vi "Get Injected Value static.vi"(8 "error in (no error)":errorcluster, 11 "Fault-Injection_SGL in":refnum<class "Fault-Injection_SGL.lvclass">) -> (0 "error out":errorcluster, 2 "Value":T1, 3 "Fault-Injection_SGL out":refnum<class "Fault-Injection_SGL.lvclass">)   [LabVIEW 2021, in "Fault-Injection_SGL.lvclass"]
uses:
  Fault-Injection_SGL.lvclass
  Value Type.ctl
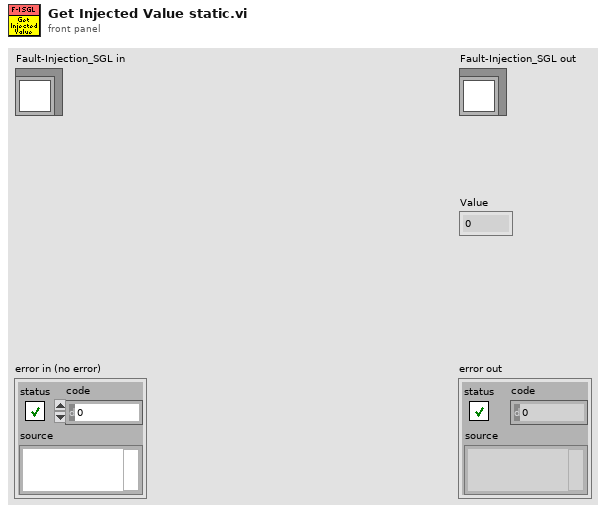
[diagram p1: front panel]
types:
  T1 = typedef "Fault-Injection_SGL.lvclass/Value Type.ctl" = sgl
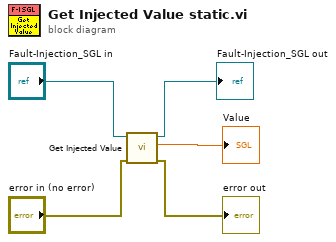
[diagram p0: block diagram]
diagram:
  n1 = call-dynamic "Get Injected Value.vi"("error in (no error)"="error in (no error)", "Fault-Injection_Boolean in"="Fault-Injection_SGL in") -> ("error out"=→"error out":errorcluster, "Value"=→"Value":T1, "Fault-Injection_Boolean out"=→"Fault-Injection_SGL out":refnum<class "Fault-Injection_SGL.lvclass">)  [unwired: 7 in]
